vi "ConnectorPaneWiring_LV2Template.vi"(0 "VI in":refnum<vi>, 11 "error in (no error)":errorcluster) -> (15 "error out":errorcluster)   [LabVIEW 2014]
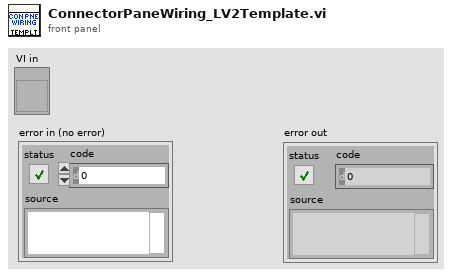
[diagram p1: front panel]
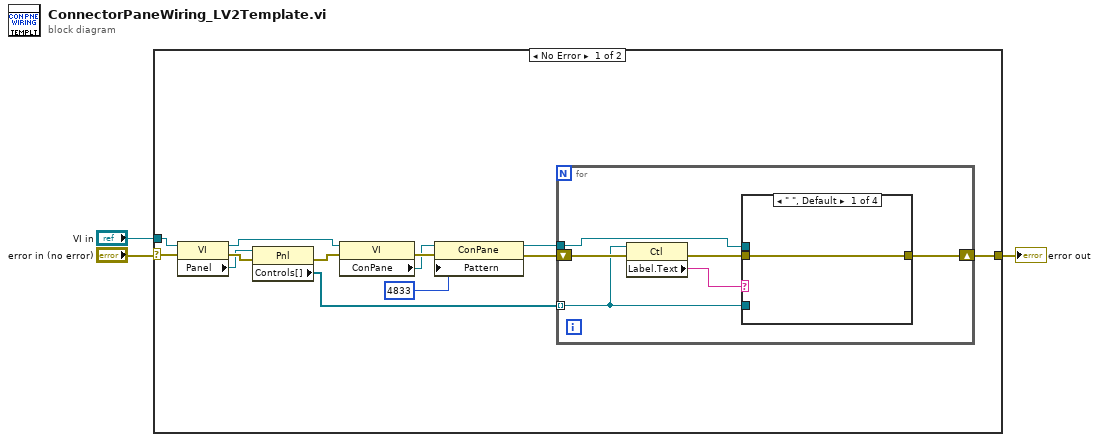
[diagram p0: block diagram]
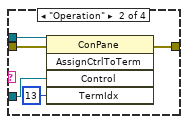
[diagram p2: hidden frame]
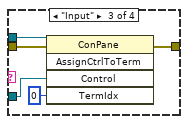
[diagram p3: hidden frame]
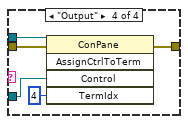
[diagram p4: hidden frame]
diagram:
  n1 = case shown="No Error" "error in (no error)" {
    selector: "error in (no error)" -> [w16 w39]
    tunnel: [w11 w39] -> w2
    tunnel: "VI in" -> [w9 _]
    frame No Error {
      n2 = property class="VI"(reference=w9, error in=w16) -> (reference out=w8:refnum<vi>, error out=w10:errorcluster, "Panel"=w6:refnum<vi>)
      n3 = property class="Pnl"(reference=w6, error in=w10) -> (error out=w7:errorcluster, "Controls[]"=w5:refnum<vi>[])  [unwired: 1 out]
      n4 = property class="VI"(reference=w8, error in=w7) -> (error out=w15:errorcluster, "ConPane"=w13:refnum<vi>)  [unwired: 1 out]
      n5 = property class="ConPane"(reference=w13, error in=w15, "Pattern"=u32 4833) -> (reference out=w4:refnum<vi>, error out=w14:errorcluster)
      n6 = for {
        shift-right: [w22] -> w11
        shift-left: w14 -> [w21]
        tunnel: w5 -> [w18] mode=indexing
        tunnel: w4 -> [w17]
        n7 = property class="Ctl"(reference=w18, error in=w21) -> (error out=w20:errorcluster, "Label.Text"=w19:string)  [unwired: 1 out]
        n8 = case shown="\" \", Default" w19 {
          tunnel: [w23 w28 w33 w38] -> w22
          tunnel: w17 -> [_ w26 w31 w36]
          tunnel: w20 -> [w23 w27 w32 w37]
          tunnel: w18 -> [_ w25 w30 w35]
          frame " ", Default {
          }
          frame "Operation" {
            n9 = invoke class="ConPane" method="AssignCtrlToTerm"(reference=w26, error in=w27, "Control"=w25, "TermIdx"=u32 13 ("Terminal Index")) -> (error out=w28:errorcluster)  [unwired: 1 in, 4 out]
          }
          frame "Input" {
            n10 = invoke class="ConPane" method="AssignCtrlToTerm"(reference=w31, error in=w32, "Control"=w30, "TermIdx"=u32 0 ("Terminal Index")) -> (error out=w33:errorcluster)  [unwired: 1 in, 4 out]
          }
          frame "Output" {
            n11 = invoke class="ConPane" method="AssignCtrlToTerm"(reference=w36, error in=w37, "Control"=w35, "TermIdx"=u32 4 ("Terminal Index")) -> (error out=w38:errorcluster)  [unwired: 1 in, 4 out]
          }
        }
      }
    }
    frame Error {
    }
  }
  "error out" <- w2
